vi "Prompt for Step--Init UI.vi"(8 "error in (no error)":errorcluster, 10 "Control Ref Map":map{string, refnum<vi>}(c390), 11 "Assertion Step in":refnum<class "Assertion Step.lvclass">) -> (0 "error out":errorcluster, 3 "Assertion Step out":refnum<class "Assertion Step.lvclass">)   [LabVIEW 2020, in "MacroAssert.lvlib" / "Assertion Step.lvclass"]
uses:
  Assertion Step.lvclass
  Step/Step.lvclass
  Assertion Step.lvclass/Assertion Step.ctl
  MacroAssert.lvlib
  Support/Get Control Reference by Label (1D STR).vi
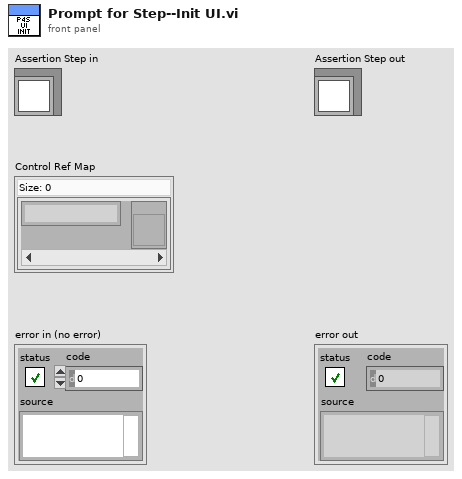
[diagram p1: front panel]
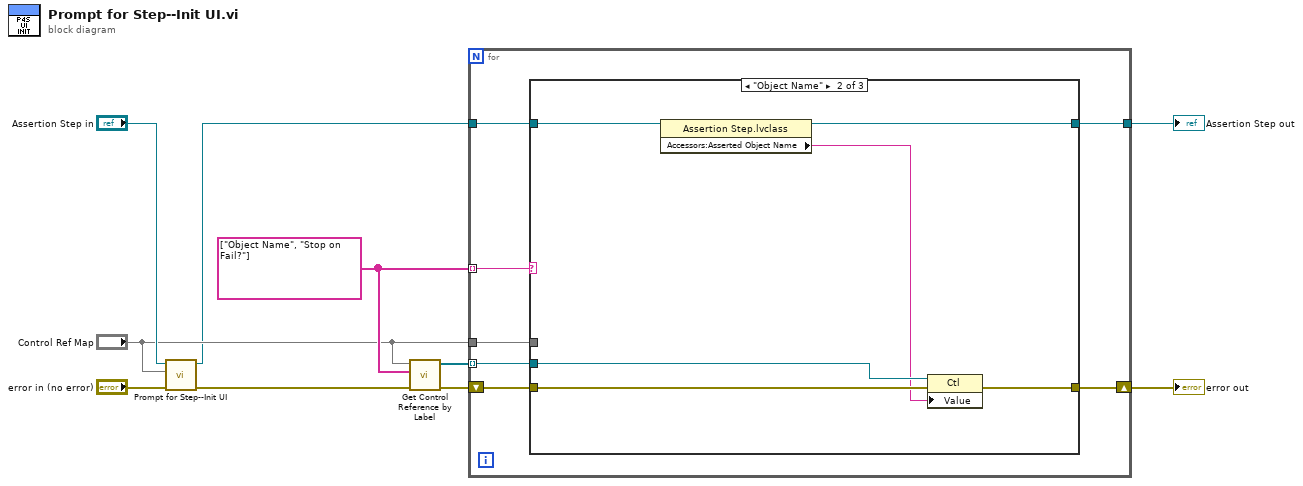
[diagram p0: block diagram]
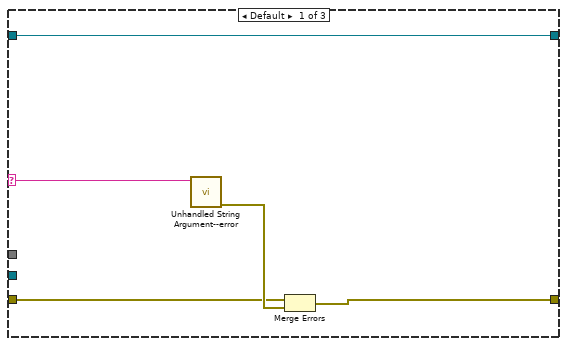
[diagram p2: hidden frame]
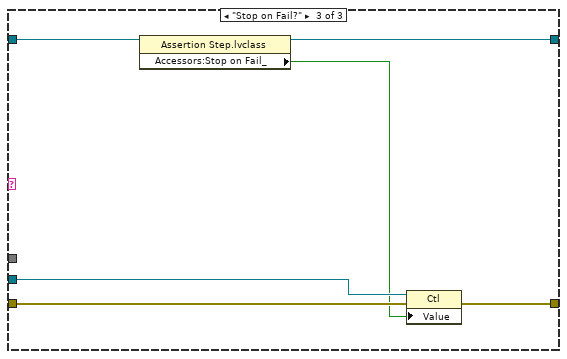
[diagram p3: hidden frame]
diagram:
  w9 = string[] ["Object Name", "Stop on Fail?"]
  n1 = call-parent "Prompt for Step--Init UI.vi"("error in (no error)"="error in (no error)", "Control Ref Map"="Control Ref Map", "Step in"="Assertion Step in") -> ("error out"=w4:errorcluster, "Step out"=w1:refnum<class "Assertion Step.lvclass">)  [unwired: 7 in]
  n2 = call-poly "Get Control Reference by Label.vi"("error in (no error)"=w4, "Control Names"=w9, "Control Ref Map"="Control Ref Map") -> ("error out"=w10:errorcluster, "Control Refs"=w8:refnum<vi>[])  [unwired: 6 in, 1 out]
  n3 = for {
    tunnel: w1 -> [w15]
    tunnel: [w13] -> w6
    tunnel: w9 -> [w16] mode=indexing
    tunnel: w8 -> [w14] mode=indexing
    shift-right: [w12] -> w5
    shift-left: w10 -> [w17]
    tunnel: "Control Ref Map" -> [w11]
    n4 = case shown="\"Object Name\"" w16 {
      selector: w16 -> [w19 _ _]
      tunnel: w17 -> [w21 w25 w31]
      tunnel: w15 -> [w18 w28 w34]
      tunnel: w14 -> [_ w26 w32]
      tunnel: [w18 w27 w33] -> w13
      tunnel: [w20 w23 w29] -> w12
      tunnel: w11 -> [_ _ _]
      frame Default {
        n5 = call "Unhandled String Argument--error.vi"("Argument"=w19) -> ("error out"=w22:errorcluster)  [unwired: 10 in]
        n6 = Merge Errors(w21, w22) -> (w20:errorcluster)
      }
      frame "Object Name" {
        n7 = property class="Assertion Step.lvclass"(reference=w28) -> (reference out=w27:refnum<class "Assertion Step.lvclass">, "Accessors:Asserted Object Name"=w24:string)  [unwired: 1 in, 1 out]
        n8 = property class="Ctl"(reference=w26, error in=w25, "Value"=w24) -> (error out=w23:errorcluster)  [unwired: 1 out]
      }
      frame "Stop on Fail?" {
        n9 = property class="Assertion Step.lvclass"(reference=w34) -> (reference out=w33:refnum<class "Assertion Step.lvclass">, "Accessors:Stop on Fail_"=w30:bool)  [unwired: 1 in, 1 out]
        n10 = property class="Ctl"(reference=w32, error in=w31, "Value"=w30) -> (error out=w29:errorcluster)  [unwired: 1 out]
      }
    }
  }
  "error out" <- w5
  "Assertion Step out" <- w6
